vi "Get Game Pad Values.vi"(8 "error in (no error)":errorcluster, 11 "Game Engine in":refnum<class "Game Engine.lvclass">) -> (0 "error out":errorcluster, 1 "Right":bool, 2 "Left":bool, 3 "Game Engine out":refnum<class "Game Engine.lvclass">, 4 "Down":bool, 5 "Rotate":bool, 6 "Start":bool)   [LabVIEW 2017, in "Game Engine.lvlib" / "Game Engine.lvclass"]
uses:
  Game Engine.lvclass
  Game Engine.lvclass/Game Engine.ctl
  Abstract Game Pad Interface/Abstract Game Pad Interface.lvclass
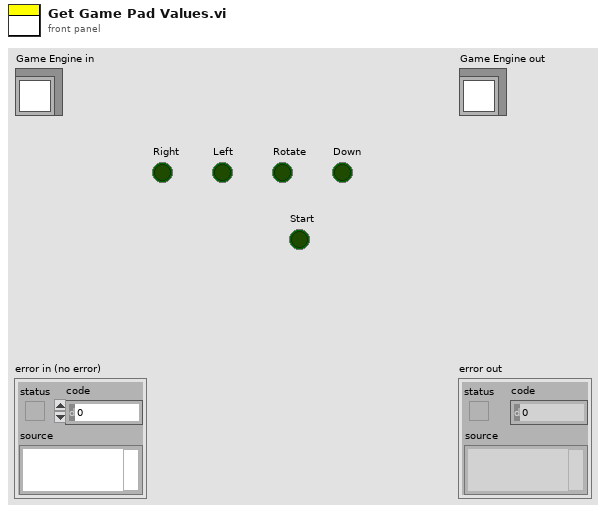
[diagram p1: front panel]
types:
  T1 = typedef "Abstract Game Pad Interface.lvclass/Game Pad Descriptor.ctl" = cluster{"Up":bool, "Down":bool, "Left":bool, "Right":bool, "A":bool, "B":bool, "Start":bool, "Select":bool}
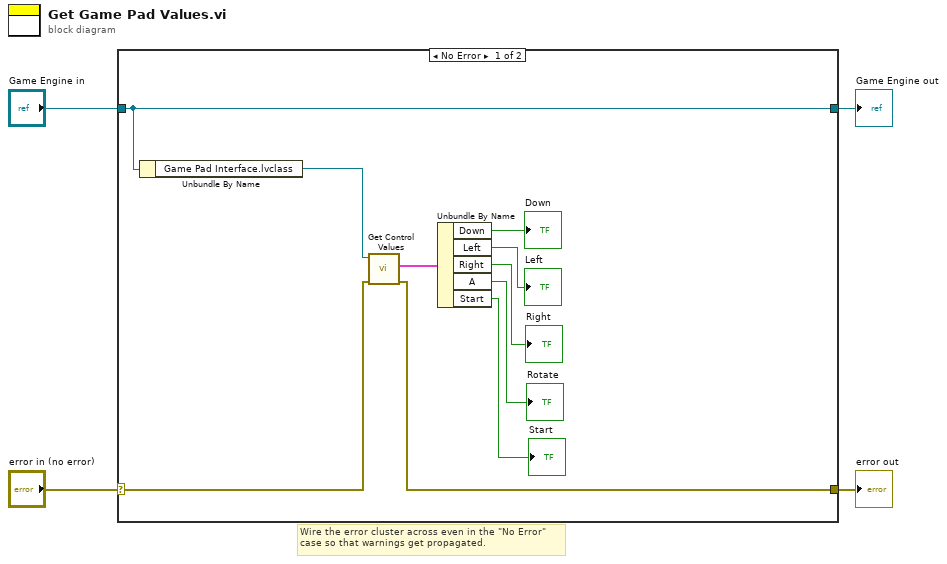
[diagram p0: block diagram]
diagram:
  # "Wire the error cluster across even in the \"No Error\"\ncase so that warnings get propagated."
  n1 = case shown="No Error" "error in (no error)" {
    selector: "error in (no error)" -> [w5 w16]
    tunnel: [w7 w16] -> w3
    tunnel: [w14 w15] -> w1
    tunnel: "Game Engine in" -> [w14 w15]
    frame No Error {
      n2 = Unbundle By Name(w14) -> ("Game Pad Interface.lvclass"=w6:refnum<class "Abstract Game Pad Interface.lvclass">)
      n3 = call-dynamic "Get Control Values.vi"("error in (no error)"=w5, "Abstract Game Pad Interface in"=w6) -> ("error out"=w7:errorcluster, "Cluster"=w13:T1)  [unwired: 7 in, 1 out]
      n4 = Unbundle By Name(w13) -> ("Down"=→"Down":bool, "Left"=→"Left":bool, "Right"=→"Right":bool, "A"=→"Rotate":bool, "Start"=→"Start":bool)
    }
    frame Error {
    }
  }
  "error out" <- w3
  "Game Engine out" <- w1
